vi "GetInterfPar.vi"(8 "ErrorIn(No Error)":errorcluster caption="entrée d'erreur (pas d'erreur)", 11 "Scan(T)":bool) -> (0 "sortie d'erreur":errorcluster, 1 "InsNameIncl":bool caption="InsNameIncluded", 2 "ScanParIncl":bool caption="ScanParIncluded", 3 "Prefixe":string, 5 "GraphConfig":i32)   [LabVIEW 2010]
uses:
  <vilib>/Utility/config.llb/Read Key (String).vi
  <vilib>/Utility/config.llb/Read Key (Boolean).vi
  <vilib>/Utility/config.llb/Read Key (I32).vi
  <vilib>/Utility/config.llb/NI_LVConfig.lvlib
panel:
  in  "DisplayName":string
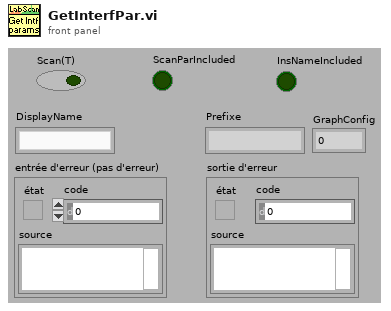
[diagram p1: front panel]
types:
  T1 = typedef "NI_LVConfig.lvlib/Config Data RefNum.ctl" = refnum<k1>
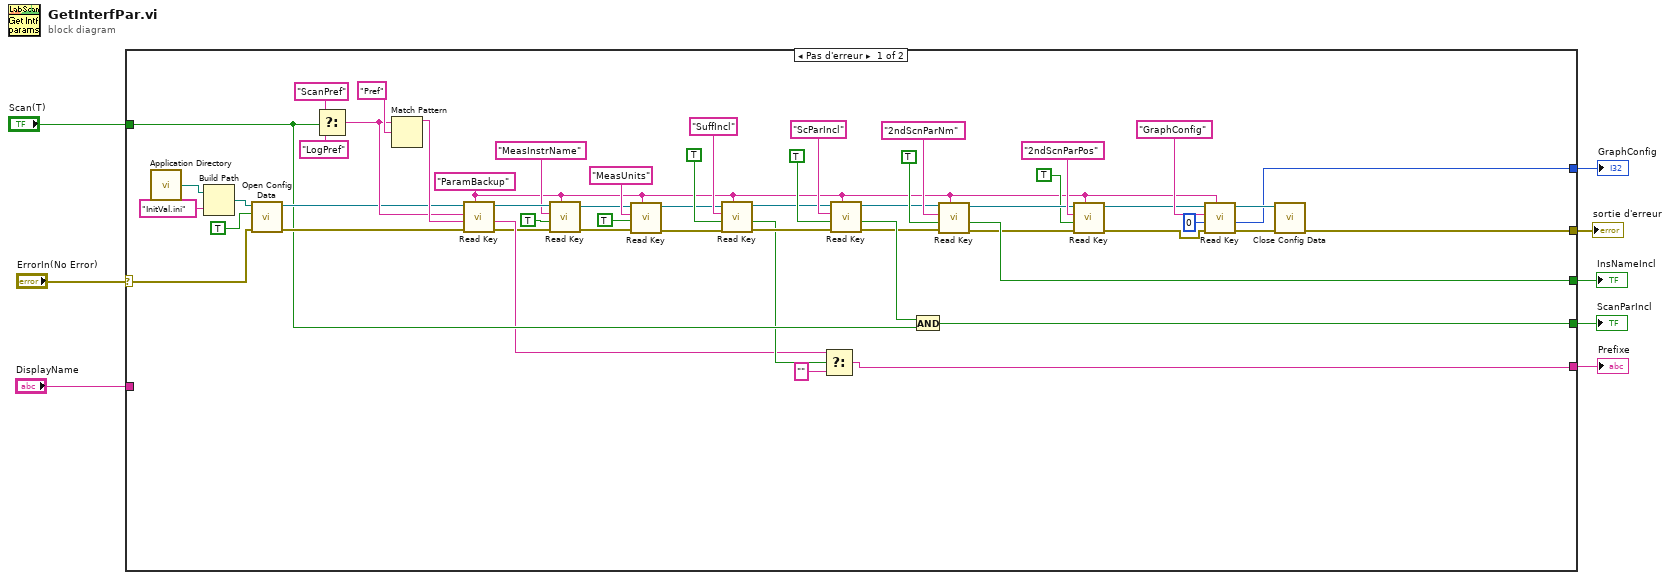
[diagram p0: block diagram]
diagram:
  n1 = case shown="Pas d'erreur" "ErrorIn(No Error)" {
    selector: "ErrorIn(No Error)" -> [w50 w62]
    tunnel: [w49 w62] -> w7
    tunnel: "Scan(T)" -> [w45 _]
    tunnel: [w31 _] -> w5
    tunnel: [w46 _] -> w4
    tunnel: [w39 _] -> w3
    tunnel: "DisplayName" -> [_ _]
    tunnel: [w16 _] -> w1
    frame No Error {
      w9 = "ParamBackup"
      n2 = call <vilib>:"Application Directory.vi"() -> ("Application Directory"=w54:path)
      n3 = Build Path(base path=w54, name or relative path="InitVal.ini") -> (appended path=w53:path)
      n4 = call <vilib>:"Open Config Data.vi"("error in (no error)"=w50, "create file if necessary (T)"=TRUE ("create file if necessary? (T)"), "configuration file path"=w53) -> ("error out"=w55:errorcluster, "refnum"=w58:T1)  [unwired: 6 in, 1 out]
      n5 = Select(t="ScanPref", s=w45, f="LogPref") -> (s? t:f=w59:string)
      n6 = Match Pattern(string=w59, regular expression="Pref") -> (before substring=w61:string)  [unwired: 1 in, 3 out]
      n7 = call-poly <vilib>:"Read Key.vi"("section"=w9, "error in (no error)"=w55, "default value"=w61, "key"=w59, "refnum"=w58) -> ("error out"=w30:errorcluster, "value"=w33:string, "refnum out"=w29:T1)  [unwired: 3 in, 1 out]
      n8 = call-poly <vilib>:"Read Key.vi"("section"=w9, "error in (no error)"=w30, "default value"=TRUE, "key"="MeasInstrName", "refnum"=w29) -> ("error out"=w25:errorcluster, "refnum out"=w22:T1)  [unwired: 3 in, 2 out]
      n9 = call-poly <vilib>:"Read Key.vi"("section"=w9, "error in (no error)"=w25, "default value"=TRUE, "key"="MeasUnits", "refnum"=w22) -> ("error out"=w24:errorcluster, "refnum out"=w21:T1)  [unwired: 3 in, 2 out]
      n10 = call-poly <vilib>:"Read Key.vi"("section"=w9, "error in (no error)"=w24, "default value"=TRUE, "key"="SuffIncl", "refnum"=w21) -> ("error out"=w35:errorcluster, "value"=w34:bool, "refnum out"=w36:T1)  [unwired: 3 in, 1 out]
      n11 = Select(t=w33, s=w34, f="" ("cas faux")) -> (s? t:f=w31:string)
      n12 = call-poly <vilib>:"Read Key.vi"("section"=w9, "error in (no error)"=w35, "default value"=TRUE, "key"="ScParIncl", "refnum"=w36) -> ("error out"=w41:errorcluster, "value"=w44:bool, "refnum out"=w40:T1)  [unwired: 3 in, 1 out]
      n13 = And(x=w44, y=w45) -> (x .and. y?=w46:bool)
      n14 = call-poly <vilib>:"Read Key.vi"("section"=w9, "error in (no error)"=w41, "default value"=TRUE, "key"="2ndScnParNm", "refnum"=w40) -> ("error out"=w14:errorcluster, "value"=w39:bool, "refnum out"=w13:T1)  [unwired: 3 in, 1 out]
      n15 = call-poly <vilib>:"Read Key.vi"("section"=w9, "error in (no error)"=w14, "default value"=TRUE ("value"), "key"="2ndScnParPos", "refnum"=w13) -> ("error out"=w11:errorcluster, "refnum out"=w12:T1)  [unwired: 3 in, 2 out]
      n16 = call-poly <vilib>:"Read Key.vi"("section"=w9, "error in (no error)"=w11, "default value"=0, "key"="GraphConfig", "refnum"=w12) -> ("error out"=w20:errorcluster, "value"=w16:i32, "refnum out"=w19:T1)  [unwired: 3 in, 1 out]
      n17 = call <vilib>:"Close Config Data.vi"("error in (no error)"=w20, "refnum"=w19) -> ("error out"=w49:errorcluster)  [unwired: 8 in, 1 out]
    }
    frame Error {
    }
  }
  "sortie d'erreur" <- w7
  "Prefixe" <- w5
  "ScanParIncl" <- w4
  "InsNameIncl" <- w3
  "GraphConfig" <- w1
